vi "Log temperatures.vi"(0 "LSC218 sensors":T1 {"Time stamp" format="%<%H:%M:%S%2u\n%Y/%m/%d>T"}, 1 "Time":timestamp, 2 "Tmp logfile in":refnum<file>, 5 "VTI":dbl, 7 "Sample":dbl, 9 "Trap":dbl, 11 "HePot":dbl, 12 "Field [T]":dbl format="%#_13g", 13 "Logging interval (10s)":dbl=10.0) -> (4 "Tmp logfile ref":refnum<file>, 6 "logInterval":bool caption="Time has Elapsed", 15 "error out":errorcluster)   [LabVIEW 2022 SP3]
uses:
  Subsystem modules/Magnet module/ctl/Cryostat temperature sensors.ctl
  Subsystem modules/Magnet module/Magnet module.lvlib
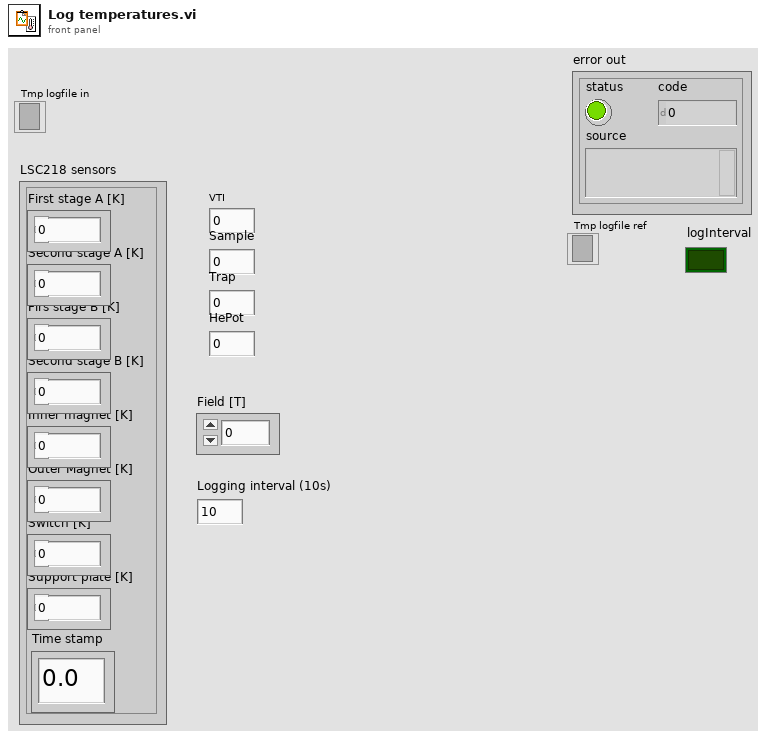
[diagram p1: front panel]
types:
  T1 = typedef "Magnet module.lvlib/Cryostat temperature sensors.ctl" = cluster{"First stage A [K]":dbl, "Second stage A [K]":dbl, "Firs stage B [K]":dbl, "Second stage B [K]":dbl, "Inner magnet [K]":dbl, "Outer Magnet [K]":dbl, "Switch [K]":dbl, "Support plate [K]":dbl, "Time stamp":dbl}
  T2 = enum16{"open", "replace", "create", "open or create", "replace or create", "replace or create with confirmation"}
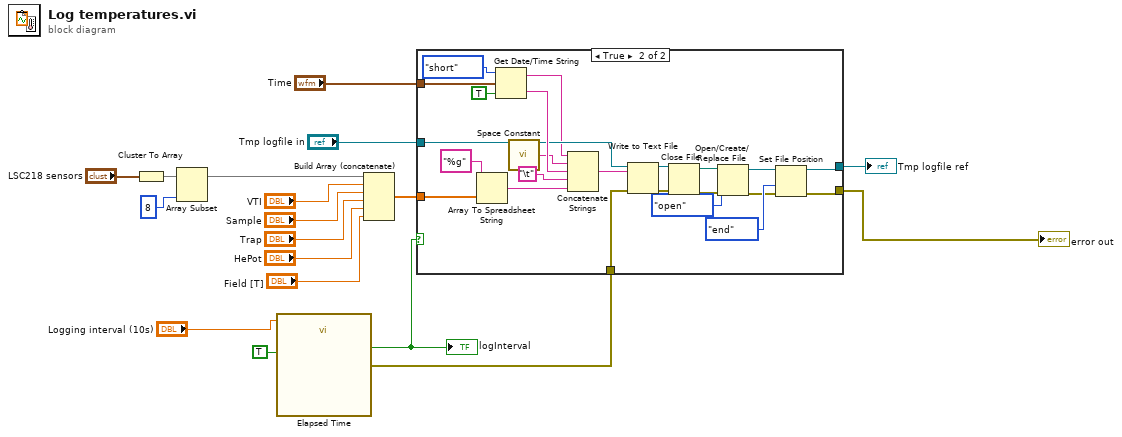
[diagram p0: block diagram]
diagram:
  n1 = Cluster To Array(cluster="LSC218 sensors") -> (array=w18:dbl[])
  n2 = Array Subset(array=w18, length=8) -> (w2:dbl[])  [unwired: 1 in]
  n3 = call "Elapsed Time"("Time Target (s)"="Logging interval (10s)", "Auto Reset"=TRUE) -> ("Time has Elapsed"=w6:bool, "error out"=w5:errorcluster)  [unwired: 10 in, 6 out]
  "logInterval" <- w6
  n4 = Build Array (concatenate)(w2, "VTI", "Sample", "Trap", "HePot", "Field [T]") -> (w14:dbl[])
  n5 = case shown="True" w6 {
    tunnel: "Time" -> [_ w40]
    tunnel: "Tmp logfile in" -> [w19 w36]
    tunnel: w14 -> [_ w34]
    tunnel: [w20 w21] -> w8
    tunnel: w5 -> [w20 w31]
    tunnel: [w19 w22] -> w3
    frame False {
    }
    frame True {
      n6 = Array To Spreadsheet String(array=w34, 3:"%g" ("format string")) -> (spreadsheet string=w43:string)  [unwired: 1 in]
      n7 = Get Date/Time String(date format (0)=enum16{"short", "long", "abbreviated"}."short", seconds (now)=w40, want seconds? (F)=TRUE) -> (date string=w33:string, time string=w38:string)
      n8 = call <vilib>:"Space Constant.vi"() -> ("String"=w32:string)
      n9 = Concatenate Strings(w33, w32, w38, "\t", w43) -> (w41:string)
      n10 = Write to Text File(file (use dialog)=w36, text=w41, error in=w31) -> (refnum out=w30:refnum<file>, error out=w29:errorcluster)  [unwired: 1 in, 1 out]
      n11 = Close File(refnum=w30, error in=w29) -> (path=w28:path, error out=w27:errorcluster)
      n12 = Open/Create/Replace File(file path (use dialog)=w28, error in=w27, operation (0:open)=T2."open") -> (refnum out=w24:refnum<file>, error out=w23:errorcluster)  [unwired: 3 in, 1 out]
      n13 = Set File Position(refnum=w24, from (0:start)=enum16{"start", "end", "current"}."end", error in=w23) -> (refnum out=w22:refnum<file>, error out=w21:errorcluster)  [unwired: 1 in]
    }
  }
  "error out" <- w8
  "Tmp logfile ref" <- w3
